vi "Target Validity Test.vi"(8 "Difference Image":T1, 11 "Particle Report":T2) -> (3 "Target is valid?":bool)   [LabVIEW 2012]
uses:
  <vilib>/vision/Image Controls.llb/IMAQ Image.ctl
  <vilib>/vision/NI_Vision_Development_Module.lvlib
panel:
  in  "Max Proportion\nof Area Filled in\nOriginal":dbl=0.5
  in  "Width vs. Height Tolerance":dbl=0.5
  in  "Actual height":dbl=18.0
  in  "Actual width":dbl=24.0
  in  "Minimum \"Rectangleness\"":dbl=0.6
  in  "Minimum Area":dbl=416.0
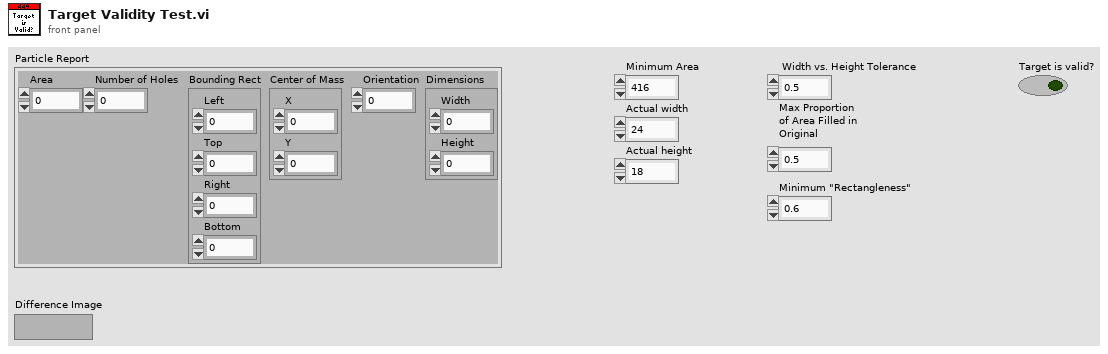
[diagram p1: front panel]
types:
  T1 = typedef "IMAQ Image.ctl" = refnum<image>
  T2 = cluster{"Area":dbl, "Number of Holes":dbl, "Bounding Rect":cluster{"Left":dbl, "Top":dbl, "Right":dbl, "Bottom":dbl}, "Center of Mass":cluster{"X":dbl, "Y":dbl}, "Orientation":dbl, "Dimensions":cluster{"Width":dbl, "Height":dbl}}
  T3 = cluster{"Left":dbl, "Top":dbl, "Right":dbl, "Bottom":dbl}
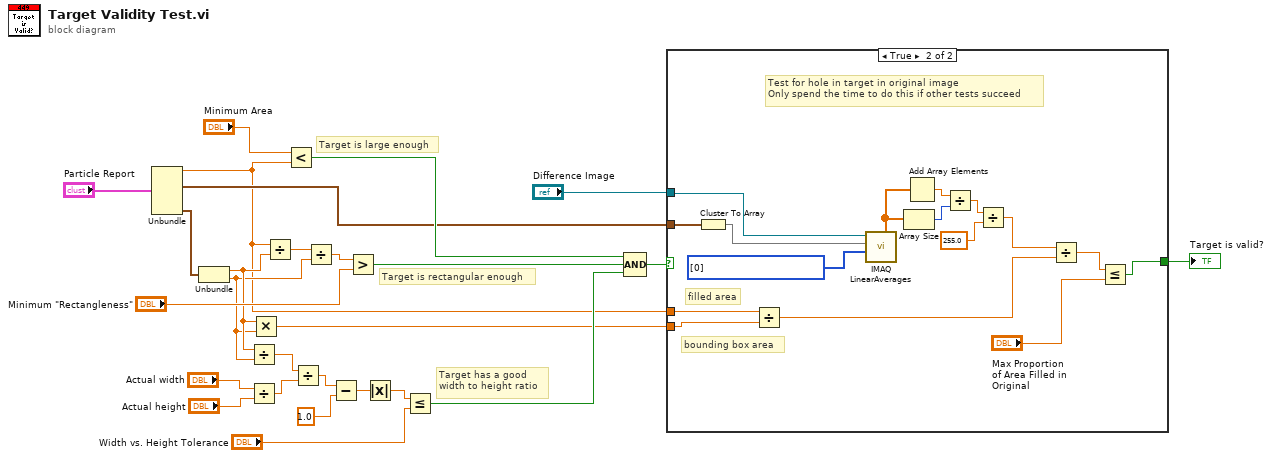
[diagram p0: block diagram]
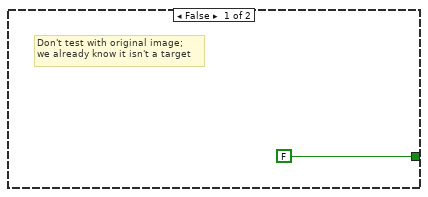
[diagram p2: hidden frame]
diagram:
  # "Target has a good \nwidth to height ratio"
  # "Target is rectangular enough"
  # "Target is large enough"
  n1 = Unbundle("Particle Report") -> ("Area"=w2:dbl, "Bounding Rect"=w6:T3, "Dimensions"=w22:cluster{"Width":dbl, "Height":dbl})  [unwired: 3 out]
  n2 = Unbundle(w22) -> ("Width"=w5:dbl, "Height"=w4:dbl)
  n3 = Divide(x=w5, y=w4) -> (x/y=w19:dbl)
  n4 = Divide(x="Actual width", y="Actual height") -> (x/y=w18:dbl)
  n5 = Multiply(x=w5, y=w4) -> (x*y=w3:dbl)
  n6 = Divide(x=w2, y=w5) -> (x/y=w23:dbl)
  n7 = Less?(x="Minimum Area", y=w2) -> (x < y?=w12:bool)
  n8 = Divide(x=w19, y=w18) -> (x/y=w16:dbl)
  n9 = Divide(x=w23, y=w4) -> (x/y=w1:dbl)
  n10 = Subtract(x=w16, y=1.0) -> (x-y=w15:dbl)
  n11 = Greater?(x=w1, y="Minimum \"Rectangleness\"") -> (0:w11:bool)
  n12 = Absolute Value(x=w15) -> (abs(x)=w14:dbl)
  n13 = Less Or Equal?(x=w14, y="Width vs. Height Tolerance") -> (x <= y?=w10:bool)
  n14 = Compound Arithmetic op=AND(w12, w11, w10) -> (w9:bool)
  n15 = case shown="True" w9 {
    tunnel: [FALSE w31] -> w8
    tunnel: "Difference Image" -> [_ w43]
    tunnel: w6 -> [_ w42]
    tunnel: w3 -> [_ w35]
    tunnel: w2 -> [_ w36]
    frame False {
      # "Don't test with original image;\nwe already know it isn't a target"
    }
    frame True {
      w40 = i32[] [0] items=["X Axis Averages", "Y Axis Averages", "X + Y Axis Averages", "X - Y Axis Averages"] ("Averages")
      # "filled area"
      # "bounding box area"
      # "Test for hole in target in original image\nOnly spend the time to do this if other tests succeed"
      n16 = Cluster To Array(cluster=w42) -> (array=w41:dbl[])
      n17 = Divide(x=w36, y=w35) -> (x/y=w34:dbl)
      n18 = call "IMAQ LinearAverages"("Averages"=w40, "Optional Rectangle"=w41, "Image Src"=w43) -> ("X Axis Averages"=w38:sgl[])  [unwired: 4 in, 4 out]
      n19 = Array Size(array=w38) -> (size(s)=w37:i32)
      n20 = Add Array Elements(numeric array=w38) -> (sum=w39:sgl)
      n21 = Divide(x=w39, y=w37) -> (x/y=w30:sgl)
      n22 = Divide(x=w30, y=sgl 255.0) -> (x/y=w28:sgl)
      n23 = Divide(x=w28, y=w34) -> (x/y=w33:dbl)
      n24 = Less Or Equal?(x=w33, y="Max Proportion\nof Area Filled in\nOriginal") -> (x <= y?=w31:bool)
    }
  }
  "Target is valid?" <- w8
